vi "gsp_simulator_setup.vi"(4 "error in (no error)":errorcluster, 5 "baud rate (57600)":u32=57600, 6 "Timeout (1000 ms)":u32=1000, 7 "VISA resource name":refnum<visa-resource-name>="ASRL2::INSTR") -> (0 "error out":errorcluster)   [LabVIEW 2015]
doc: "Sets the serial port up for Silvermax communication. The stop character is 0x0D = 13."
uses:
  <vilib>/Instr/_visa.llb/VISA Configure Serial Port (Instr).vi
  gsp_simulator_global.vi
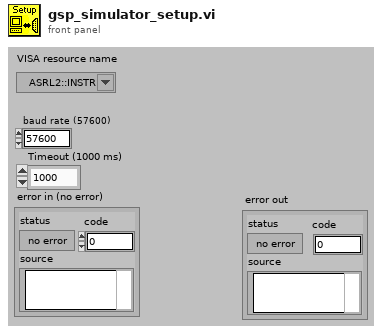
[diagram p1: front panel]
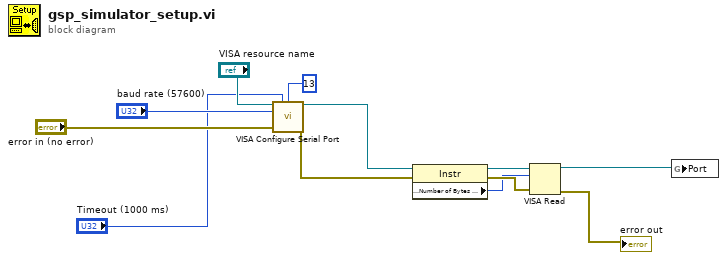
[diagram p0: block diagram]
diagram:
  n1 = call-poly "VISA Configure Serial Port"("VISA resource name"="VISA resource name", "timeout (10sec)"="Timeout (1000 ms)", "termination char\n(0xA = '\\n' = LF)"=u8 13 ("termination char\n(0xA = '\\n' = LF)"), "baud rate (9600)"="baud rate (57600)", "error in (no error)"="error in (no error)") -> ("VISA resource name out"=w8:refnum<visa-resource-name>, "error out"=w7:errorcluster)  [unwired: 9 in]
  n2 = property class="Instr"(reference=w8, error in=w7) -> (reference out=w6:refnum<visa-resource-name>, error out=w5:errorcluster, "Serial Settings:Number of Bytes at Serial Port"=w4:u32)
  n3 = VISA Read(VISA resource name=w6, byte count=w4, error in (no error)=w5) -> (VISA resource name out=w3:refnum<visa-resource-name>, error out=→"error out":errorcluster)  [unwired: 2 out]
  n4 = global write "gsp_simulator_global.vi" "Port"(w3) -> ()
